vi "DAQ Analog Write.vi"(8 "error in (no error)":errorcluster, 10 "Outputs":dbl[](array[numeric]), 11 "Refnum in":refnum<k21>) -> (0 "error out":errorcluster, 3 "Refnum out":refnum<k21>)   [LabVIEW 2016]
uses:
  <vilib>/DAQmx/write.llb/DAQmx Write (Analog 1D DBL NChan 1Samp).vi
  <vilib>/DAQmx/miscellaneous.llb/DAQmx Fill In Error Info.vi
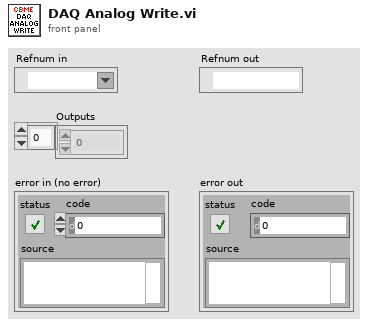
[diagram p1: front panel]
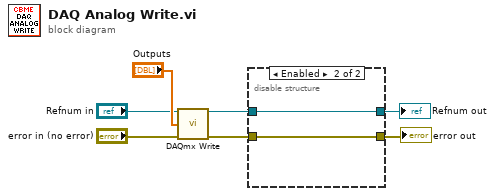
[diagram p0: block diagram]
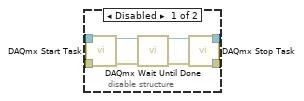
[diagram p2: hidden frame]
diagram:
  n1 = call-poly <vilib>:"DAQmx Write.vi"("task/channels in"="Refnum in", "data"="Outputs", "error in"="error in (no error)") -> ("task out"=w4:refnum<k21>, "error out"=w3:errorcluster)  [unwired: 10 in, 1 out]
  n2 = disable-structure shown="Enabled" {
    disable-tunnel: w4 -> [w15 w17]
    disable-tunnel: w3 -> [w14 w16]
    disable-tunnel: [w9 w17] -> w2
    disable-tunnel: [w8 w16] -> w1
    frame Disabled {
      n3 = call <vilib>:"DAQmx Start Task.vi"("task/channels in"=w15, "error in"=w14) -> ("task out"=w13:refnum<k21>, "error out"=w12:errorcluster)  [unwired: 12 in]
      n4 = call <vilib>:"DAQmx Wait Until Done.vi"("task/channels in"=w13, "error in"=w12) -> ("task out"=w11:refnum<k21>, "error out"=w10:errorcluster)  [unwired: 12 in]
      n5 = call <vilib>:"DAQmx Stop Task.vi"("task/channels in"=w11, "error in"=w10) -> ("task out"=w9:refnum<k21>, "error out"=w8:errorcluster)  [unwired: 12 in]
    }
    frame Enabled {
    }
  }
  "error out" <- w1
  "Refnum out" <- w2
